vi "Climber_Notifier_Begin.vi"   [LabVIEW 2020]
uses:
  Subsystems/Climber/Climber_Control_States.ctl
  Subsystems/Climber/Climber_Cluster.ctl
  Globals/Climber_Globals.vi
types:
  T1 = typedef "Climber_Cluster.ctl" = cluster{"Control_State":T2, "Outer_Arm_Pivot_Throttle":dbl, "Outer_Arm_Elevator_Throttle":dbl, "Inner_Arm_Pivot_Throttle":dbl, "Enable_Climber_Sequence":bool}
  T2 = typedef "Climber_Control_States.ctl" = enum16{"No-Op", "Manual_%Vbus", "Climbing_Sequence"}
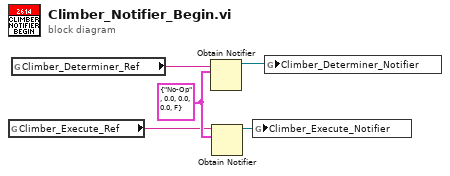
[diagram p0: block diagram]
diagram:
  w3 = T1 {"Control_State"=enum."No-Op", "Outer_Arm_Pivot_Throttle"=0.0, "Outer_Arm_Elevator_Throttle"=0.0, "Inner_Arm_Pivot_Throttle"=0.0, "Enable_Climber_Sequence"=FALSE}
  n1 = global read "Climber_Globals.vi" "Climber_Execute_Ref"() -> (w2:string)
  n2 = global read "Climber_Globals.vi" "Climber_Determiner_Ref"() -> (w1:string)
  n3 = Obtain Notifier(name (unnamed)=w1, notification data type=w3) -> (notifier out=w5:refnum<notifier>)  [unwired: 2 in, 2 out]
  n4 = Obtain Notifier(name (unnamed)=w2, notification data type=w3) -> (notifier out=w4:refnum<notifier>)  [unwired: 2 in, 2 out]
  n5 = global write "Climber_Globals.vi" "Climber_Execute_Notifier"(w4) -> ()
  n6 = global write "Climber_Globals.vi" "Climber_Determiner_Notifier"(w5) -> ()
